vi "_jsonDecodeKafkaMessage.vi"() -> ()   [LabVIEW 2019]
uses:
  KafkaLVLib/API/KafkaConsumerEvent.ctl
panel:
  in  "Message":cluster{"Key":string, "value":T1[]}
  out "error out":errorcluster
  in  "error in (no error)":errorcluster
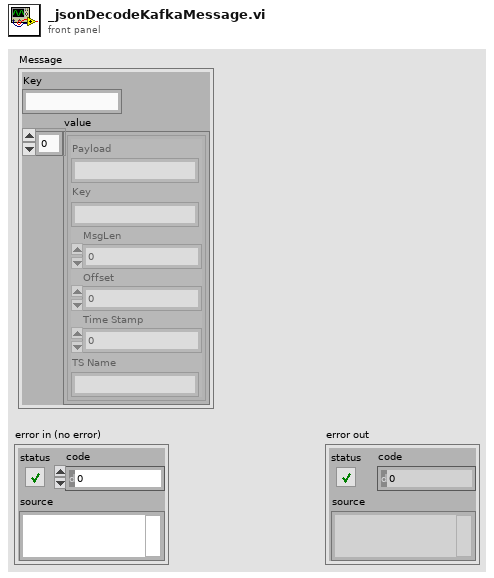
[diagram p1: front panel]
types:
  T1 = typedef "KafkaConsumerEvent.ctl" = cluster{"Payload":string, "Key":string, "MsgLen":u64, "Offset":i64, "Time Stamp":i64, "TS Name":string}
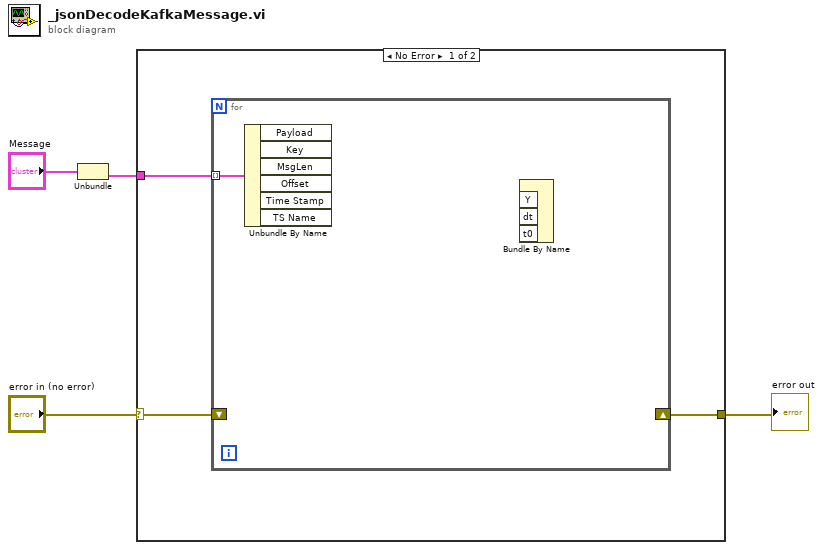
[diagram p0: block diagram]
diagram:
  n1 = Unbundle("Message") -> ("value"=w2:T1[])  [unwired: 1 out]
  n2 = case shown="No Error" "error in (no error)" {
    selector: "error in (no error)" -> [w6 w9]
    tunnel: w2 -> [w7 _]
    tunnel: [w5 w9] -> w1
    frame No Error {
      n3 = for {
        tunnel: w7 -> [w8] mode=indexing
        shift-right: [_] -> w5
        shift-left: w6 -> [_]
        n4 = Unbundle By Name(w8) -> ()  [unwired: 6 out]
        n5 = Bundle By Name() -> ()  [unwired: 4 in, 1 out]
      }
    }
    frame Error {
    }
  }
  "error out" <- w1
